vi "GetControlRef.vi"(6 "Case Sensitive? (TRUE)":bool=TRUE, 8 "error in (no error)":errorcluster, 9 "Indicator (F=Control)":bool, 10 "Control Name":string, 11 "VI Refnum":refnum<vi>) -> (0 "error out":errorcluster, 1 "Found?":bool, 2 "Ctl Refnum":refnum<vi>)   [LabVIEW 2011, in "VITesterUtilities.lvlib"]
uses:
  Libraries/VITesterUtilities.lvlib
  <userlib>/_OpenG.lib/appcontrol/appcontrol.llb/Close Generic Object Refnum (Array)__ogtk.vi
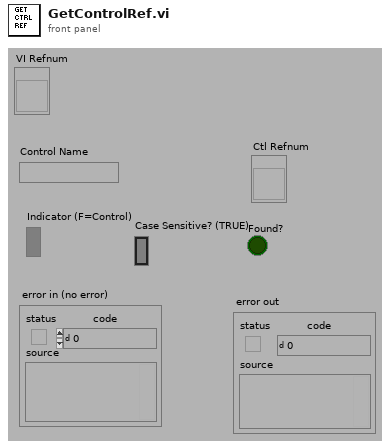
[diagram p1: front panel]
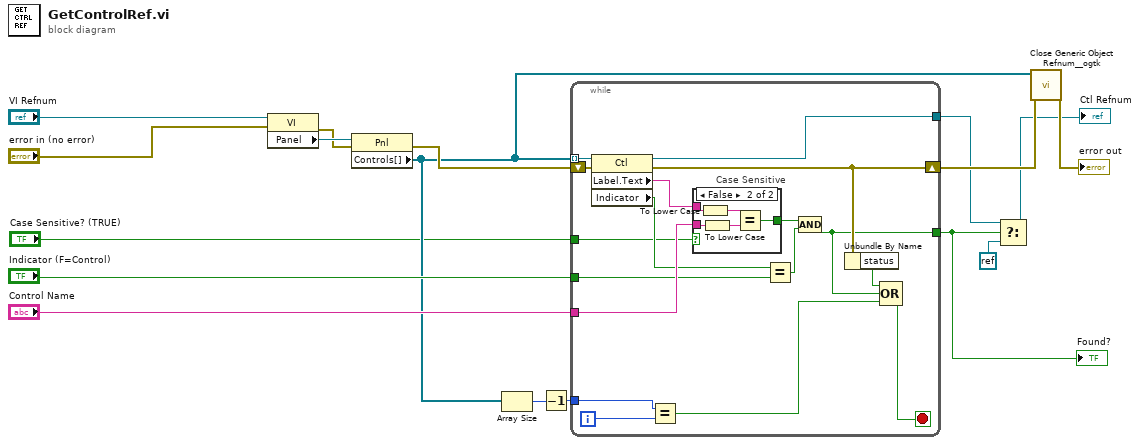
[diagram p0: block diagram]
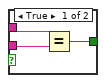
[diagram p2: hidden frame]
diagram:
  n1 = property class="VI"(reference="VI Refnum", error in="error in (no error)") -> (error out=w12:errorcluster, "Panel"=w16:refnum<vi>)  [unwired: 1 out]
  n2 = property class="Pnl"(reference=w16, error in=w12) -> (error out=w13:errorcluster, "Controls[]"=w8:refnum<vi>[])  [unwired: 1 out]
  n3 = Array Size(array=w8) -> (size(s)=w11:i32)
  n4 = Decrement(x=w11) -> (x-1=w10:i32)
  n5 = while {
    tunnel: w8 -> [w34] mode=indexing
    tunnel: "Control Name" -> [w32]
    tunnel: "Indicator (F=Control)" -> [w30]
    shift-right: [w25] -> w7
    shift-left: w13 -> [w27]
    tunnel: [w26] -> w2
    tunnel: w10 -> [w22]
    tunnel: [w19] -> w5
    tunnel: "Case Sensitive? (TRUE)" -> [w18]
    i -> [w23]
    stop <- w20 stop-if-true
    n6 = property class="Ctl"(reference=w34, error in=w27) -> (reference out=w26:refnum<vi>, error out=w25:errorcluster, "Label.Text"=w33:string, "Indicator"=w31:bool)
    n7 = Equal?(x=w22, y=w23) -> (x = y?=w21:bool)
    n8 = case "Case Sensitive" shown="False" w18 {
      tunnel: w33 -> [w37 w42]
      tunnel: w32 -> [w36 w41]
      tunnel: [w35 w40] -> w29
      frame True {
        n9 = Equal?(x=w37, y=w36) -> (x = y?=w35:bool)
      }
      frame False {
        n10 = To Lower Case(string=w42) -> (all lower case string=w39:string)
        n11 = To Lower Case(string=w41) -> (all lower case string=w38:string)
        n12 = Equal?(x=w39, y=w38) -> (x = y?=w40:bool)
      }
    }
    n13 = Equal?(x=w31, y=w30) -> (x = y?=w28:bool)
    n14 = Compound Arithmetic op=AND(w29, w28) -> (w19:bool)
    n15 = Unbundle By Name(w25) -> ("status"=w24:bool)
    n16 = Compound Arithmetic op=OR(w24, w19, w21) -> (w20:bool)
  }
  "Found?" <- w5
  n17 = Select(t=w2, s=w5, f=refnum<k0> refnum) -> (s? t:f=→"Ctl Refnum":refnum<vi>)
  n18 = call-poly <userlib>:"Close Generic Object Refnum__ogtk.vi"("error in (no error)"=w7, "Gen Refnum Array"=w8) -> ("error out"=→"error out":errorcluster)  [unwired: 9 in]
